vi "main_init_panel.vi"(5 "Running?":refnum<vi>, 6 "Reset":refnum<vi>, 7 "Auto Scroll":refnum<vi>, 8 "Break Button":refnum<vi>, 9 "Pause Button":refnum<vi>, 10 "Stop Button":refnum<vi>, 11 "Run":refnum<vi>) -> ()   [LabVIEW 2019]
panel:
  # "*******************************************************************\nBiogas Plant Control\n\nAuthor: Paul Zügel\nGCSC-Frankfurt am Main 2020\n\n*******************************************************************"
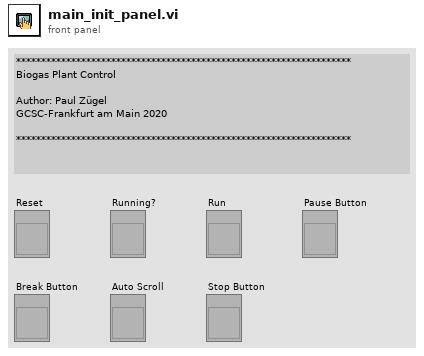
[diagram p1: front panel]
types:
  T1 = enum8{"Enabled", "Disabled", "Disabled and Grayed Out"}
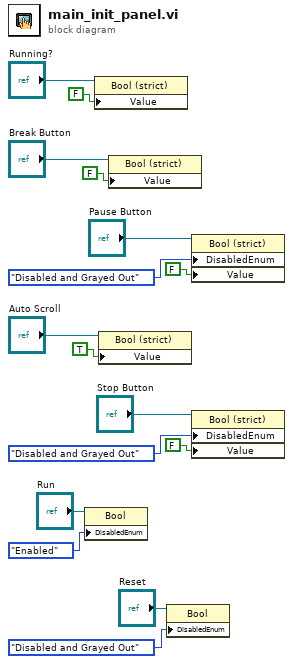
[diagram p0: block diagram]
diagram:
  n1 = property on="Property Node" class="Bool"(reference="Run", "DisabledEnum"=T1."Enabled" ("Disabled")) -> ()  [unwired: 1 in, 2 out]
  n2 = property class="Bool (strict)"(reference="Running?", "Value"=FALSE) -> ()  [unwired: 1 in, 2 out]
  n3 = property on="Property Node" class="Bool (strict)"(reference="Auto Scroll", "Value"=TRUE ("Auto Scroll")) -> ()  [unwired: 1 in, 2 out]
  n4 = property class="Bool (strict)"(reference="Break Button", "Value"=FALSE) -> ()  [unwired: 1 in, 2 out]
  n5 = property on="Property Node" class="Bool"(reference="Reset", "DisabledEnum"=T1."Disabled and Grayed Out" ("Disabled")) -> ()  [unwired: 1 in, 2 out]
  n6 = property on="Property Node" class="Bool (strict)"(reference="Pause Button", "DisabledEnum"=T1."Disabled and Grayed Out" ("Disabled"), "Value"=FALSE ("Stop Button")) -> ()  [unwired: 1 in, 2 out]
  n7 = property on="Property Node" class="Bool (strict)"(reference="Stop Button", "DisabledEnum"=T1."Disabled and Grayed Out" ("Disabled"), "Value"=FALSE ("Pause Button")) -> ()  [unwired: 1 in, 2 out]
